vi "DTW.vi"(8 "Reference Sequence":T1, 11 "Test Sequence":T1) -> (1 "Cost":dbl)   [LabVIEW 2013]
uses:
  <vilib>/silver_ctls/ArrayMatrixCluster/Real Matrix NI_Silver.ctl
  <vilib>/imath/engines/lvmath2/RunTimeEngine/ErrorHandling/NIMS_Finalize Error.vi
  <vilib>/imath/engines/lvmath2/RunTimeEngine/IndexRead/NIMS M(S,S).vi
  <instcachedir>/0/NIMS M(S,S)_AC51E74150A542F7991B9634C66F3096.lvgen/NIMS M(S,S)_AC51E74150A542F7991B9634C66F3096_000.vi
  <vilib>/imath/engines/lvmath2/RunTimeEngine/IndexReplace/NIMS M(S,S)=S.vi
  <instcachedir>/0/NIMS M(S,S)=S_EC2A86BD47664E68AE45685B0A86CA9E.lvgen/NIMS M(S,S)=S_EC2A86BD47664E68AE45685B0A86CA9E_000.vi
  <vilib>/imath/engines/lvmath2/RunTimeEngine/ErrorHandling/NIMS_Create Error From Enums.vi
  <vilib>/imath/engines/lvmath2/RunTimeEngine/RangeToken/NIMS_Range_R2 - Integer.vi
  <instcachedir>/0/NIMS_Range_R2 - Integer_C51C130E5EA5464EA148B28CDAB9615A.lvgen/NIMS_Range_R2 - Integer_C51C130E5EA5464EA148B28CDAB9615A_000.vi
  <vilib>/imath/engines/lvmath2/RunTimeEngine/NodeEndStatement/NIMS_NodeEndStatement_Output.vi
  <instcachedir>/0/NIMS_NodeEndStatement_Output_53EC0D466D134D7ABD903AC30B43404B.lvgen/NIMS_NodeEndStatement_Output_53EC0D466D134D7ABD903AC30B43404B_001.vi
  <vilib>/imath/engines/lvmath2/RunTimeEngine/CommandStatement/MC_CommandStatement_break.vi
  <vilib>/imath/engines/lvmath2/RunTimeEngine/BuiltInFunctions/min/1 input/NIMS_min(RV).vi
  <instcachedir>/0/NIMS_min(RV)_EE2DD3E2888846108C5160A664B67832.lvgen/NIMS_min(RV)_EE2DD3E2888846108C5160A664B67832_000.vi
  <vilib>/imathl/engines/lvmath/Functions/Error Handling/Create Error.vi
panel:
  out "Local Cost Matrix":dbl[][](array[numeric])
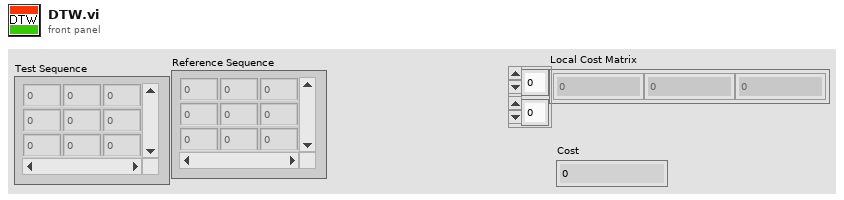
[diagram p1: front panel]
types:
  T1 = typedef "Real Matrix NI_Silver.ctl" = dbl[][]
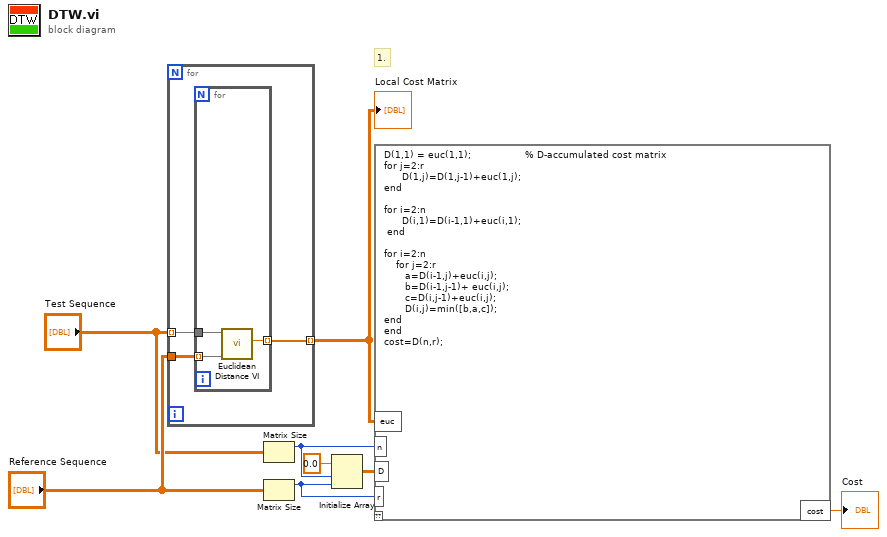
[diagram p0: block diagram]
diagram:
  # "1."
  n1 = for {
    tunnel: "Test Sequence" -> [w10] mode=indexing
    tunnel: "Reference Sequence" -> [w11]
    tunnel: [w9] -> w4 mode=indexing
    n2 = for {
      tunnel: w11 -> [w13] mode=indexing
      tunnel: w10 -> [w14]
      tunnel: [w12] -> w9 mode=indexing
      n3 = call "Euclidean Distance VI.vi"("Reference"=w13, "Test"=w14) -> ("Dist"=w12:dbl)  [unwired: 9 in]
    }
  }
  "Local Cost Matrix" <- w4
  n4 = Matrix Size(0:"Test Sequence") -> (1:w5:i32)  [unwired: 1 out]
  n5 = Matrix Size(0:"Reference Sequence") -> (1:w3:i32)  [unwired: 1 out]
  n6 = Initialize Array(0.0 ("element"), w5, w3) -> (w1:dbl[][])
  n7 = mathscript code="D(1,1) = euc(1,1);                  % D-accumulated cost matrix\nfor j=2:r\n      D(1,j)=D(1,j-1)+euc(1,j);\nend\n\nfor i=2:n\n      D(i,1)=D(i-1,1)+euc(i,1);\n end\n\nfor i=2:n\n    for j=2:r     \n       a=D(i-1,j)+euc(i,j);\n       b=D(i-1,j-1)+ euc(i,j);\n       c=D(i,j-1)+euc(i,j);\n       D(i,j)=min([b,a,c]);\nend\nend\ncost=D(n,r);"("euc"=w4, "n"=w5, "r"=w3, "D"=w1) -> ("cost"=→"Cost":dbl)  [unwired: 1 in, 1 out]
